vi "UserData_GetRS485Address.vi"(4 "Fehler (Eingang)":errorcluster caption="error out", 7 "VISA resource name in":refnum<visa-resource-name>) -> (0 "Fehler (Ausgang)":errorcluster, 2 "Address":u8, 3 "VISA resource name out":refnum<visa-resource-name>)   [LabVIEW 2018, in "JULABO DeviceDriver.lvlib"]
uses:
  JULABO DeviceDriver.lvlib
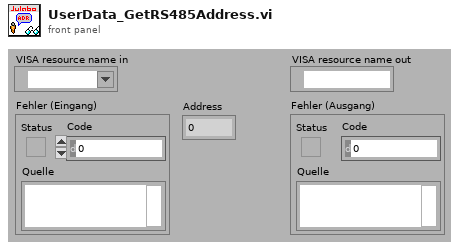
[diagram p1: front panel]
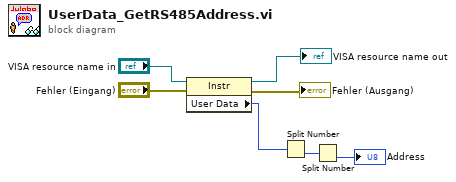
[diagram p0: block diagram]
diagram:
  n1 = property class="Instr"(reference="VISA resource name in", error in="Fehler (Eingang)") -> (reference out=→"VISA resource name out":refnum<visa-resource-name>, error out=→"Fehler (Ausgang)":errorcluster, "User Data"=w5:u32)
  n2 = Split Number(x=w5) -> (lo(x)=w4:u16)  [unwired: 1 out]
  n3 = Split Number(x=w4) -> (lo(x)=→"Address":u8)  [unwired: 1 out]
